vi "Slew Rate Demo.vi"() -> ()   [LabVIEW 2015]
panel:
  in  "Units / Second 2":dbl
  in  "Initial Output 2":dbl
  out "Slew Rate Controlled 2":bool
  out "Output 2":dbl(slide) scale=-1.0..1.0
  in  "Input 2":dbl(slide) scale=-1.0..1.0
  in  "Units / Second":dbl
  in  "Initial Output":dbl
  out "Slew Rate Controlled":bool
  out "Output":dbl(slide) scale=-1.0..1.0
  in  "Input":dbl(slide) scale=-1.0..1.0
  in  "stop":bool
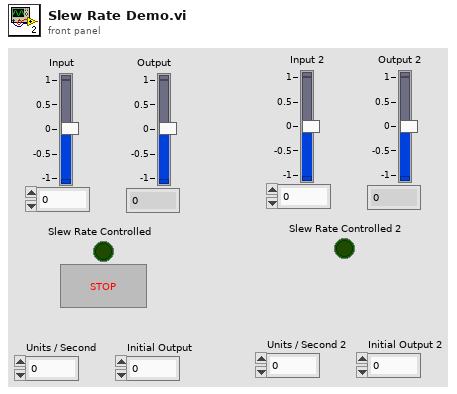
[diagram p1: front panel]
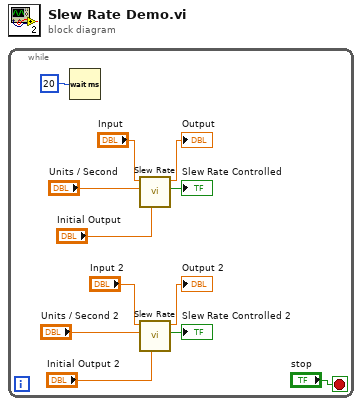
[diagram p0: block diagram]
diagram:
  n1 = while {
    stop <- "stop" stop-if-true
    n2 = Wait (ms)(milliseconds to wait=u32 20) -> ()  [unwired: 1 out]
    n3 = call "Slew Rate.vi"("Initial Output"="Initial Output", "Units / Second"="Units / Second", "Input"="Input") -> ("Slew Controlled"=→"Slew Rate Controlled":bool, "Output"=→"Output":dbl)  [unwired: 6 in, 1 out]
    n4 = call "Slew Rate.vi"("Initial Output"="Initial Output 2", "Units / Second"="Units / Second 2", "Input"="Input 2") -> ("Slew Controlled"=→"Slew Rate Controlled 2":bool, "Output"=→"Output 2":dbl)  [unwired: 6 in, 1 out]
  }
